vi "F_BSTv2.vi"() -> ()   [LabVIEW 2023]
uses:
  <vilib>/userDefined/High Color/IMAQdx.ctl
  <vilib>/MakerHub/LINX/Public/Peripherals/Digital/Digital Write 1 Chan.vi
  <vilib>/MakerHub/LINX/Public/Peripherals/PWM/PWM Set Duty Cycle 1 Chan.vi
  <vilib>/MakerHub/LINX/Public/Peripherals/Digital/Digital Write N Chans.vi
  <vilib>/MakerHub/LINX/Private/Local IO/LinxDigitalWrite.vi
  <vilib>/MakerHub/LINX/Public/Utilities/Check Channel.vi
  <vilib>/MakerHub/LINX/Public/Utilities/Open Serial.vi
  <vilib>/MakerHub/LINX/Private/Utilties/Generate Error.vi
  <vilib>/MakerHub/LINX/Public/Peripherals/PWM/PWM Set Duty Cycle N Chans.vi
  <vilib>/MakerHub/LINX/LMH-LINX.lvlib
  <vilib>/vision/driver/NI_Vision_Acquisition_Software.lvlib
  <instrlib>/MEDAQLib/MEDAQLib.lvlib
panel:
  in  "Use this stop button to end the test":bool
  in  "?":enum32{"Test Configuration", "Graph"}(tab)
  in  "Click photos in the interval of below cycles":dbl
  in  "Frequency of impact":dbl(knob) step=0.01 scale=0.0..1.0
  in  "No of Cycles":dbl
  in  "Upper limit of duty cycle (%)":dbl(slide) step=0.05 scale=0.0..100.0
  out "Device Name":string
  in  "Serial Port":refnum<visa-resource-name>="N/A"
  in  "Session In":T1
  in  "Images File Path":path
  out "IFM Error Out":string
  in  "Dutycycle File Path":path
  in  "Displacement File Path":path
  out "Image Acquisition Error Out":errorcluster
  out "Serial Communication Error Out":errorcluster
  in  "Force File Path":path
  out "No. of test cycles of dutycycle data saved":dbl
  out "No. of test cycles completed":dbl
  out "Savinng Data":u8(slide) scale=0.0..100.0
  in  "?":bool
  out "?":dbl[](graph)
  out "Right Magnet":dbl
  out "?":waveform(dbl)[](graph)
  out "Left Magnet":dbl
  out "Left Magnet 2":dbl
  out "Right Magnet 2":dbl
  out "?":waveform(dbl)[](graph)
  out "Photo clicked":bool
  out "?":T2(plugin-control)
  out "Test Progress":u8(slide) scale=0.0..100.0
  out "Left magnet max force":dbl
  out "Right magnet max force":dbl
  out "No. of test cycles of displacement data saved":dbl
  out "Savinng Data":u8(slide) scale=0.0..100.0
  in  "?":bool
  # "FBST"
  # "1 - COM PORT OF THE CONTROLLER"
  # "2 - FREQUENCY OF THE SHEAR STRESS"
  # "3 - AMPLITUDE OF THE STRESS"
  # "4 - CYCLES OF THE TEST RUN"
  # "5 - PICTURE DATA SETTINGS"
  # "DUTYCYCLE"
  # "FORCE"
  # "DISPLACEMENT"
  # "VIDEO STREAM"
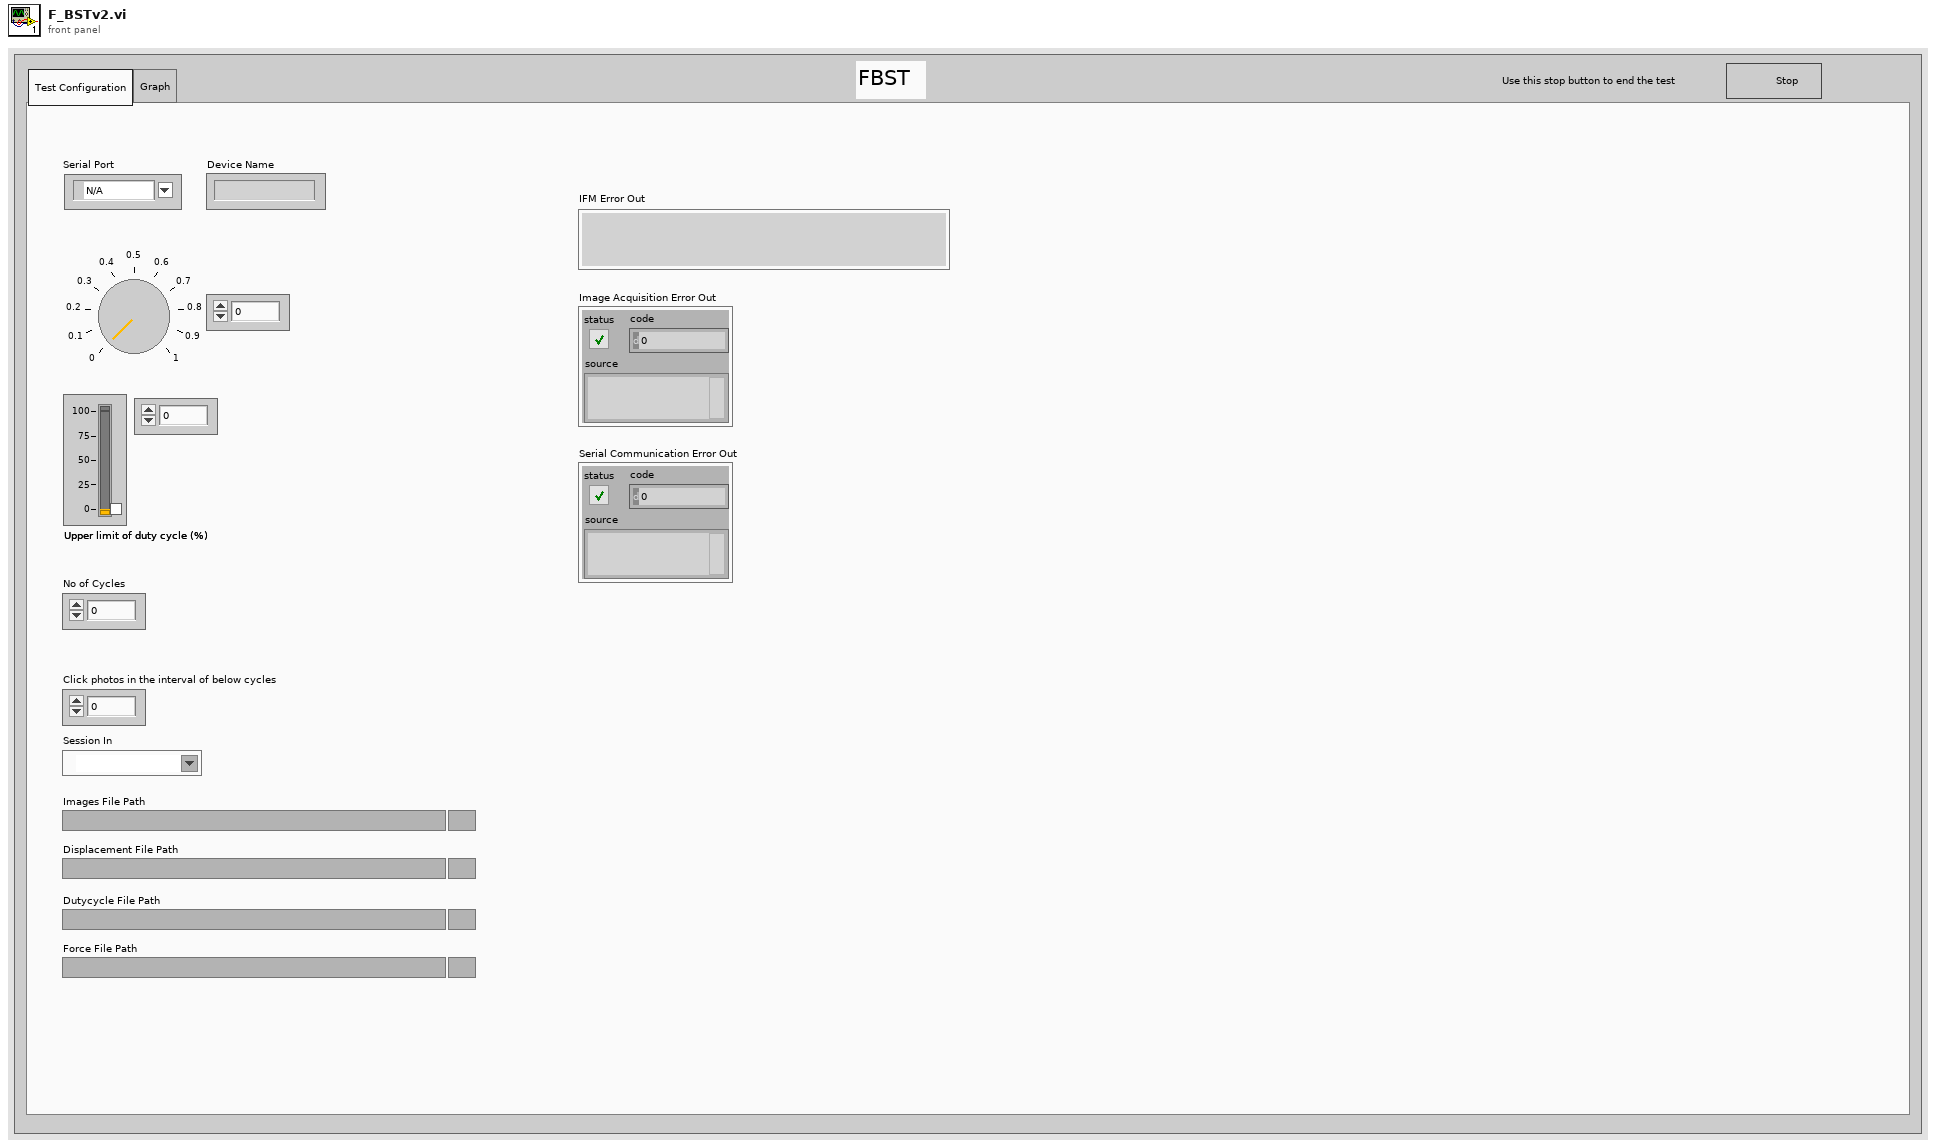
[diagram p1: front panel]
types:
  T1 = typedef "IMAQdx.ctl" = refnum<k21>
  T2 = typedef "IMAQ Image.ctl" = refnum<image>
  T3 = typedef "LMH-LINX.lvlib/LINX Ref.ctl" = cluster{"IO":T4, "Interface":T5, "LINX Device Config":T6}
  T4 = typedef "LMH-LINX.lvlib/Platform.ctl" = enum16{"Remote", "Local"}
  T5 = typedef "LMH-LINX.lvlib/Interface.ctl" = enum16{"Serial", "TCP"}
  T6 = typedef "LMH-LINX.lvlib/Device.lvlib/LINX Device Config.ctl" = cluster{"Interface":T5, "COM Port":refnum<visa-resource-name>, "TCP Configuration":T7, "Device Family":u8, "Device ID":u8, "Device Name":string, "TCP Ref":refnum<k5>, "Channels":T8}
  T7 = typedef "LMH-LINX.lvlib/Device.lvlib/TCP Config.ctl" = cluster{"IP Address":string, "Port":u16}
  T8 = typedef "LMH-LINX.lvlib/Channels.ctl" = cluster{"DI":u8[], "DO":u8[], "AI":u8[], "AO":u8[], "PWM":u8[], "QE":u8[], "UART":u8[], "I2C 2":u8[], "SPI":u8[], "CAN":u8[], "Servo":u8[], "AI Ref (V)":dbl, "AI Resolution (Bits)":u8, "AO Ref (V)":dbl, "AO Resolution (Bits)":u8}
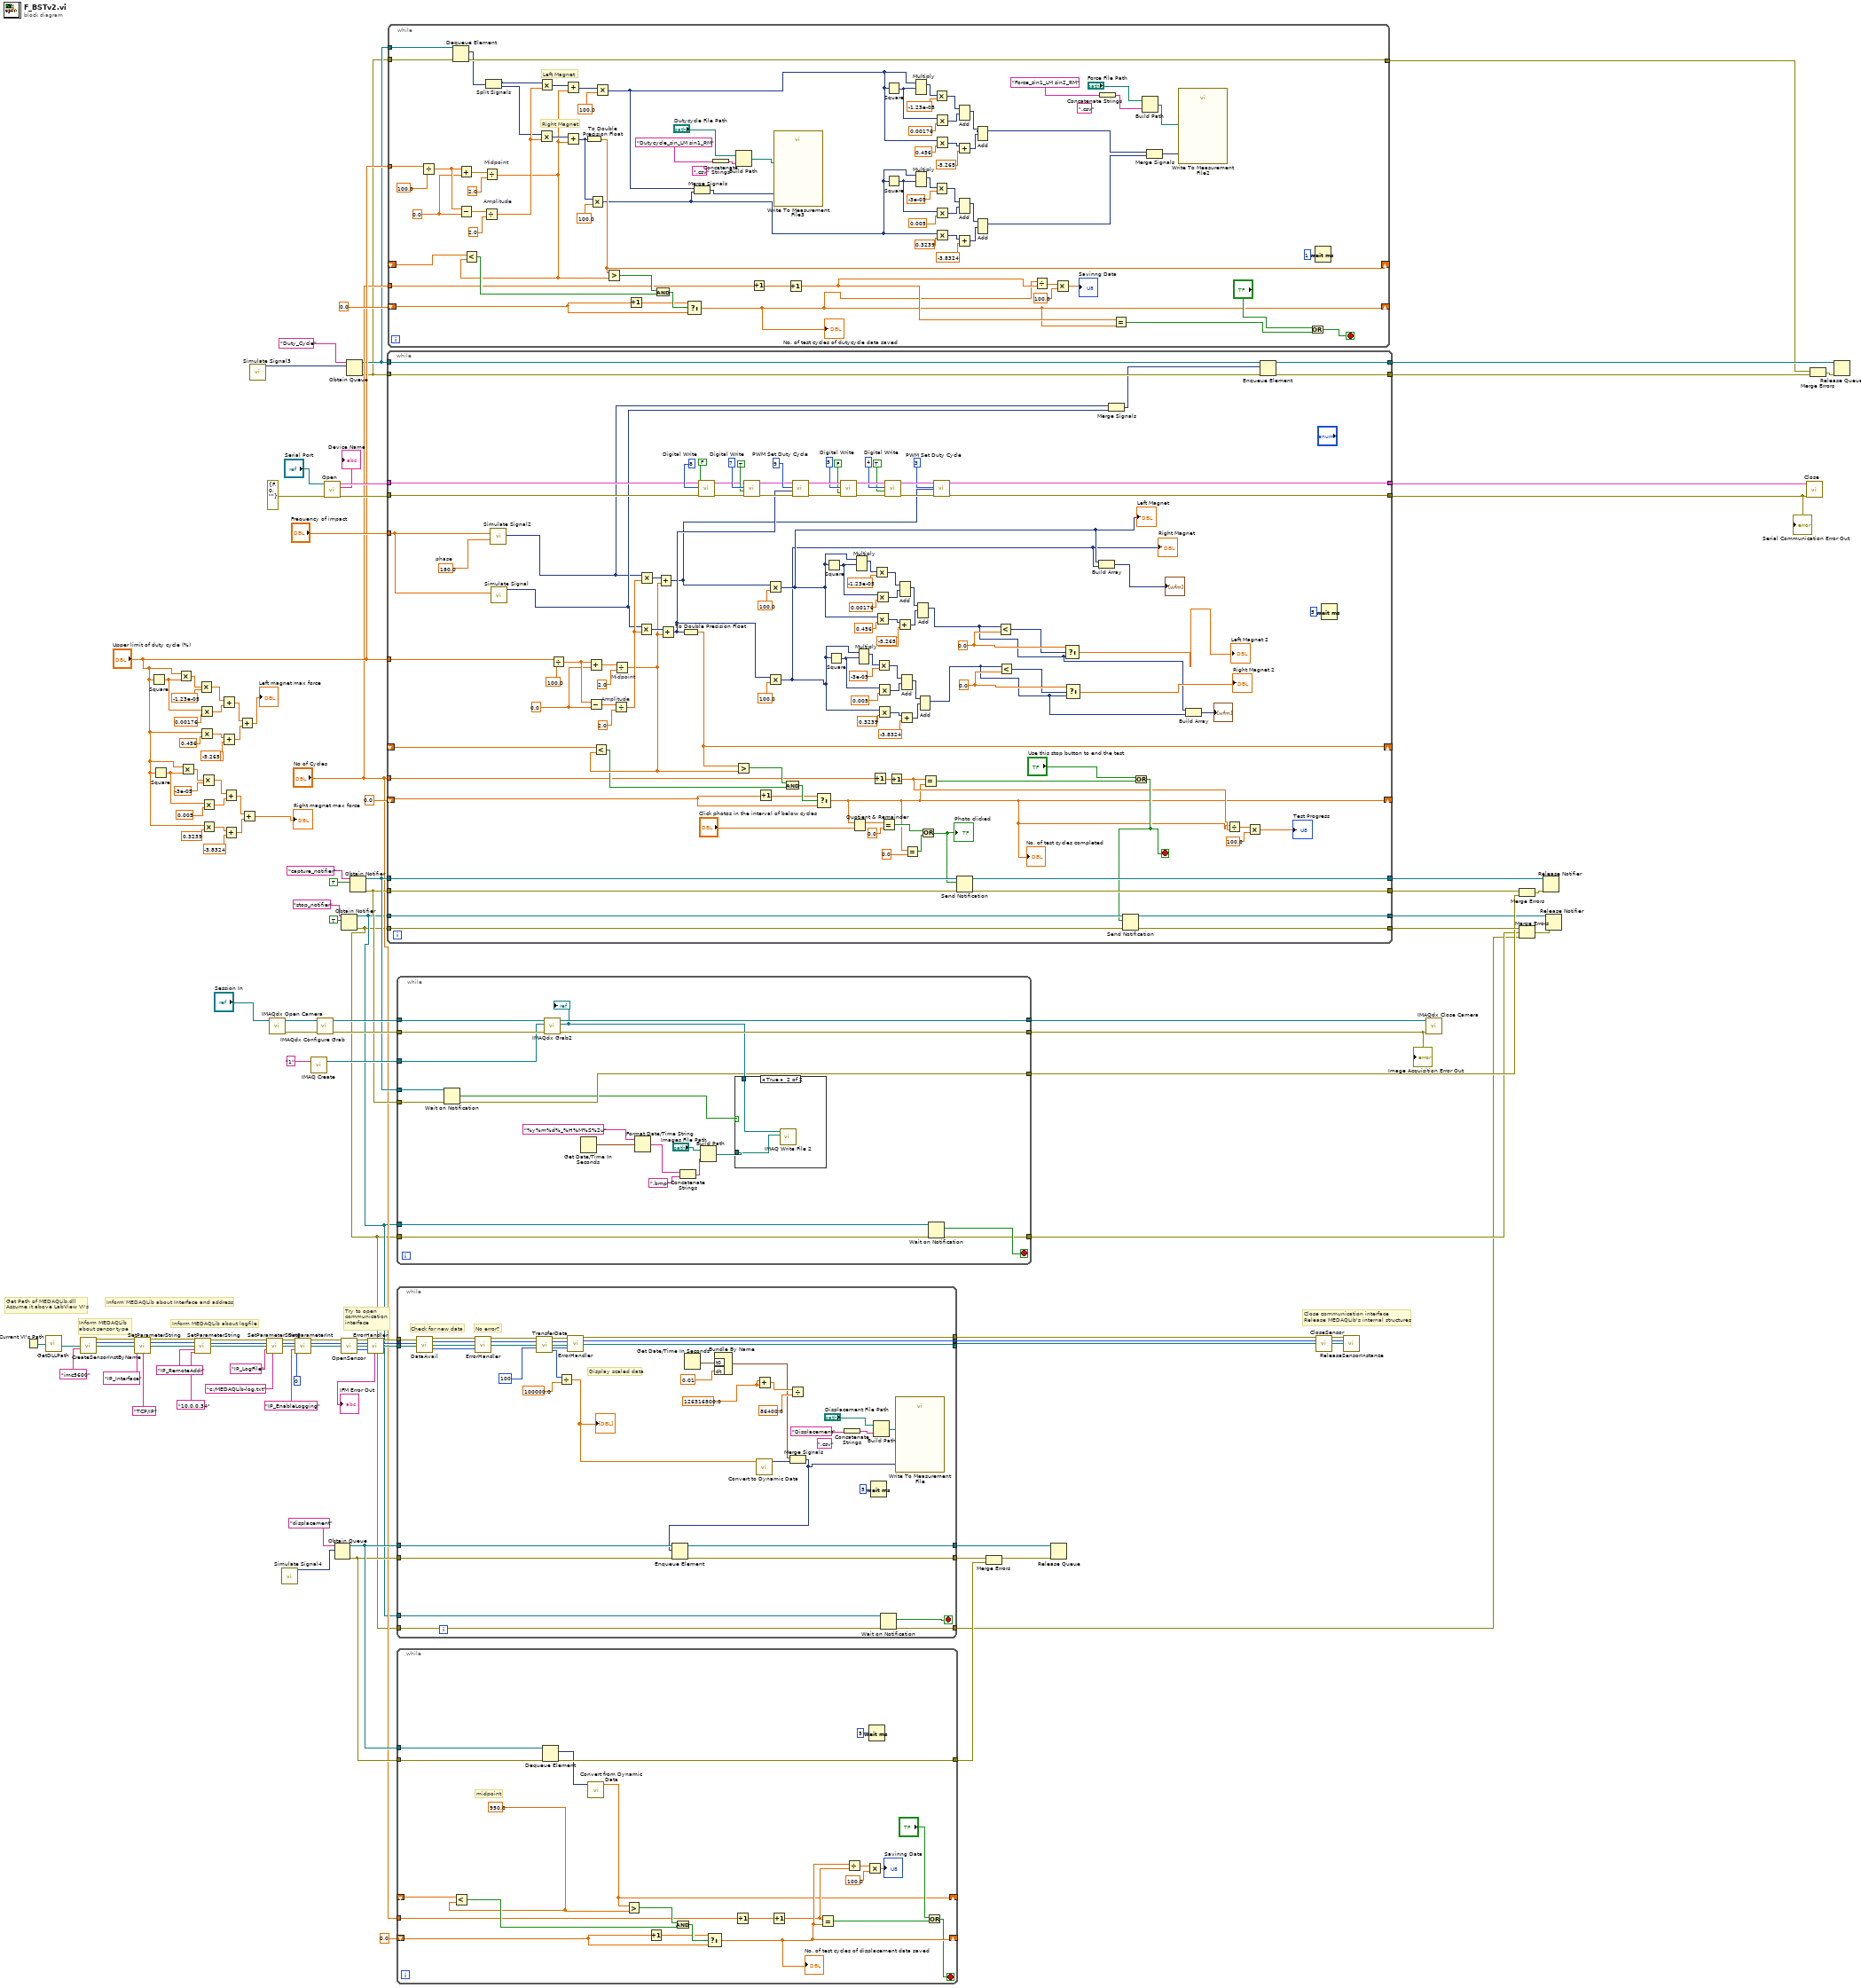
[diagram p0: block diagram]
diagram:
  (unwired) -5.265
  # "Inform MEDAQLib\nabout sensor type"
  # "Get Path of MEDAQLib.dll\nAssume it above LabView VI's"
  # "Try to open\ncommunication\ninterface"
  # "Inform MEDAQLib about logfile"
  # "Inform MEDAQLib about Interface and address"
  # "Close communication interface\nRelease MEDAQLib's internal structures"
  n1 = Current VI's Path() -> (path=w51:path)
  n2 = call <instrlib>:"GetDLLPath.vi"("VI-Path"=w51) -> ("DLL-Path"=w50:path)  [unwired: 10 out]
  n3 = call <instrlib>:"CreateSensorInstByName.vi"("DLL-Path"=w50, "sensor"="imc5600") -> ("Fehler (Ausgang)"=w47:errorcluster, "instanceHandle"=w48:u32, "DLL-Path"=w49:path)  [unwired: 1 in, 10 out]
  n4 = call <instrlib>:"SetParameterString.vi"("Fehler (Eingang, kein Fehler)"=w47, "instanceHandle"=w48, "DLL-Path"=w49, "paramName"="IP_Interface", "paramValue"="TCP/IP") -> ("Fehler (Ausgang)"=w43:errorcluster, "instanceHandle"=w42:u32, "DLL-Path"=w41:path)  [unwired: 8 out]
  n5 = Square(x="Upper limit of duty cycle (%)") -> (x^2=w33:dbl)
  n6 = Square(x="Upper limit of duty cycle (%)") -> (x^2=w22:dbl)
  n7 = Multiply(x="Upper limit of duty cycle (%)", y=w33) -> (x*y=w36:dbl)
  n8 = Multiply(x="Upper limit of duty cycle (%)", y=w22) -> (x*y=w25:dbl)
  n9 = call <instrlib>:"SetParameterString.vi"("Fehler (Eingang, kein Fehler)"=w43, "instanceHandle"=w42, "DLL-Path"=w41, "paramName"="IP_RemoteAddr", "paramValue"="10.0.0.34") -> ("Fehler (Ausgang)"=w85:errorcluster, "instanceHandle"=w84:u32, "DLL-Path"=w83:path)  [unwired: 8 out]
  n10 = Multiply(x=w36, y=-1.23e-05) -> (x*y=w31:dbl)
  n11 = Multiply(x=w33, y=0.00176) -> (x*y=w30:dbl)
  n12 = Multiply(x="Upper limit of duty cycle (%)", y=0.456) -> (x*y=w29:dbl)
  n13 = Multiply(x=w25, y=-3e-05) -> (x*y=w20:dbl)
  n14 = Multiply(x=w22, y=0.005) -> (x*y=w19:dbl)
  n15 = Multiply(x="Upper limit of duty cycle (%)", y=0.3239) -> (x*y=w18:dbl)
  n16 = Add(x=w31, y=w30) -> (x+y=w27:dbl)
  n17 = Add(x=w29, y=-5.265) -> (x+y=w26:dbl)
  n18 = Add(x=w20, y=w19) -> (x+y=w16:dbl)
  n19 = Add(x=w18, y=-3.8324) -> (x+y=w15:dbl)
  n20 = Add(x=w27, y=w26) -> (x+y=→"Left magnet max force":dbl)
  n21 = Add(x=w16, y=w15) -> (x+y=→"Right magnet max force":dbl)
  n22 = call "Simulate Signal3"() -> ("Sine"=w53:dynamicdata)  [unwired: 14 in, 1 out]
  n23 = call <instrlib>:"SetParameterString.vi"("Fehler (Eingang, kein Fehler)"=w85, "instanceHandle"=w84, "DLL-Path"=w83, "paramName"="IP_LogFile", "paramValue"="c:/MEDAQLib-log.txt") -> ("Fehler (Ausgang)"=w80:errorcluster, "instanceHandle"=w79:u32, "DLL-Path"=w78:path)  [unwired: 8 out]
  n24 = call <vilib>:"IMAQdx Open Camera.vi"("Session In"="Session In") -> ("error out"=w100:errorcluster, "Session Out"=w101:T1)  [unwired: 9 in]
  n25 = call "Simulate Signal4"() -> ("Sine"=w1:dynamicdata)  [unwired: 14 in, 1 out]
  n26 = call <instrlib>:"SetParameterInt.vi"("Fehler (Eingang, kein Fehler)"=w80, "instanceHandle"=w79, "DLL-Path"=w78, "paramName"="IP_EnableLogging", "paramValue"=0) -> ("Fehler (Ausgang)"=w75:errorcluster, "instanceHandle"=w74:u32, "DLL-Path"=w73:path)  [unwired: 8 out]
  n27 = call "IMAQ Create"("Image Name"="1") -> ("New Image"=w96:T2)  [unwired: 4 in, 1 out]
  n28 = call <vilib>:"IMAQdx Configure Grab.vi"("error in"=w100, "Session In"=w101) -> ("error out"=w97:errorcluster, "Session Out"=w98:T1)  [unwired: 8 in]
  n29 = call-poly <vilib>:"Open.vi"("Error In"=errorcluster {"status"=FALSE, "code"=0, "source"=""}, "Serial Port"="Serial Port") -> ("Error Out"=w116:errorcluster, "Device Name"=→"Device Name":string, "LINX Resource"=w117:T3)  [unwired: 7 in]
  n30 = Obtain Queue(name (unnamed)="displacement", element data type=w1) -> (queue out=w12:refnum<queue>, error out=w11:errorcluster)  [unwired: 3 in, 1 out]
  n31 = Obtain Notifier(name (unnamed)="stop_notifier", notification data type=TRUE) -> (notifier out=w4:refnum<notifier>, error out=w3:errorcluster)  [unwired: 2 in, 1 out]
  n32 = call <instrlib>:"OpenSensor.vi"("Fehler (Eingang, kein Fehler)"=w75, "instanceHandle"=w74, "DLL-Path"=w73) -> ("Fehler (Ausgang)"=w71:errorcluster, "instanceHandle"=w70:u32, "DLL-Path"=w69:path, "ERR_CODE"=w72:i32)  [unwired: 9 out]
  n33 = Obtain Queue(name (unnamed)="Duty_Cycle", element data type=w53) -> (queue out=w6:refnum<queue>, error out=w5:errorcluster)  [unwired: 3 in, 1 out]
  n34 = Obtain Notifier(name (unnamed)="capture_notifier", notification data type=TRUE) -> (notifier out=w91:refnum<notifier>, error out=w90:errorcluster)  [unwired: 2 in, 1 out]
  n35 = call <instrlib>:"ErrorHandler.vi"("Fehler (Eingang, kein Fehler)"=w71, "instanceHandle"=w70, "DLL-Path"=w69, "ERR_CODE"=w72) -> ("Fehler (Ausgang)"=w67:errorcluster, "instanceHandle"=w66:u32, "DLL-Path"=w65:path, "errText"=→"IFM Error Out":string)  [unwired: 8 out]
  n36 = while {
    tunnel: w117 -> [w205]
    tunnel: w116 -> [w235]
    tunnel: [w199] -> w115
    tunnel: [w198] -> w114
    shift-right: [w160] -> _
    shift-left: 0.0 -> [w182]
    shift-right: [w178] -> _
    shift-left: _ -> [w204]
    tunnel: w91 -> [w196]
    tunnel: [w195] -> w111
    tunnel: w90 -> [w194]
    tunnel: [w193] -> w105
    tunnel: w4 -> [w186]
    tunnel: [w185] -> w61
    tunnel: w3 -> [w174]
    tunnel: [w184] -> w104
    tunnel: w6 -> [w172]
    tunnel: w5 -> [w171]
    tunnel: [w175] -> w58
    tunnel: [w170] -> w60
    tunnel: "No of Cycles" -> [w168]
    tunnel: "Upper limit of duty cycle (%)" -> [w167]
    tunnel: "Frequency of impact" -> [w166]
    stop <- w180 stop-if-true
    w127 = 0.0 ("y")
    w130 = 0.0 ("y")
    (unwired) -5.265
    w176 = 0.0 ("y")
    w181 = 180.0  # phase
    n37 = call "Simulate Signal2"("Frequency"=w166, "Phase"=w181) -> ("Sine"=w120:dynamicdata)  [unwired: 12 in, 1 out]
    n38 = call "Simulate Signal"("Frequency"=w166) -> ("Sine"=w161:dynamicdata)  [unwired: 13 in, 1 out]
    n39 = Divide(x=w167, y=100.0) -> (x/y=w208:dbl)
    n40 = Add(x=w208, y=w176) -> (x+y=w214:dbl)
    n41 = Subtract(x=w208, y=w176) -> (x-y=w212:dbl)
    n42 = Divide "Amplitude"(x=w212, y=2.0) -> (x/y=w206:dbl)
    n43 = Divide "Midpoint"(x=w214, y=2.0) -> (x/y=w203:dbl)
    n44 = Less?(x=w204, y=w203) -> (x < y?=w201:bool)
    n45 = Multiply(x=w161, y=w206) -> (x*y=w210:dynamicdata)
    n46 = Multiply(x=w120, y=w206) -> (x*y=w207:dynamicdata)
    n47 = Add(x=w207, y=w203) -> (x+y=w144:dynamicdata)
    n48 = Add(x=w210, y=w203) -> (x+y=w145:dynamicdata)
    n49 = To Double Precision Float(number=w145) -> (double precision float=w178:dbl)
    n50 = call-poly <vilib>:"Digital Write.vi"("Error In"=w235, "Output Value"=FALSE, "DO Channel"=u8 8, "LINX Resource"=w205) -> ("Error Out"=w230:errorcluster, "LINX Resource"=w231:T3)  [unwired: 6 in]
    n51 = Greater?(x=w178, y=w203) -> (0:w202:bool)
    n52 = call-poly <vilib>:"Digital Write.vi"("Error In"=w230, "Output Value"=TRUE, "DO Channel"=u8 7, "LINX Resource"=w231) -> ("Error Out"=w226:errorcluster, "LINX Resource"=w227:T3)  [unwired: 6 in]
    n53 = Increment(x=w182) -> (x+1=w197:dbl)
    n54 = Multiply(x=w144, y=100.0) -> (x*y=w143:dynamicdata)
    "Left Magnet" <- w143
    n55 = Multiply(x=w145, y=100.0) -> (x*y=w131:dynamicdata)
    "Right Magnet" <- w131
    n56 = And(x=w202, y=w201) -> (x .and. y?=w200:bool)
    n57 = call-poly <vilib>:"PWM Set Duty Cycle.vi"("Error In"=w226, "Duty Cycle (0-1)"=w145, "PWM Channel"=u8 9, "LINX Resource"=w227) -> ("Error Out"=w220:errorcluster, "LINX Resource"=w221:T3)  [unwired: 6 in]
    n58 = Select(t=w197, s=w200, f=w182) -> (s? t:f=w160:dbl)
    "No. of test cycles completed" <- w160
    n59 = Square(x=w143) -> (x^2=w154:dynamicdata)
    n60 = Square(x=w131) -> (x^2=w139:dynamicdata)
    n61 = call-poly <vilib>:"Digital Write.vi"("Error In"=w220, "Output Value"=FALSE, "DO Channel"=u8 5, "LINX Resource"=w221) -> ("Error Out"=w223:errorcluster, "LINX Resource"=w222:T3)  [unwired: 6 in]
    n62 = Quotient & Remainder(x=w160, y="Click photos in the interval of below cycles") -> (x-y*floor(x/y)=w192:dbl)  [unwired: 1 out]
    n63 = Multiply(1:w154, 2:w143) -> (0:w157:dynamicdata)  [unwired: 1 in, 1 out]
    n64 = Multiply(1:w139, 2:w131) -> (0:w142:dynamicdata)  [unwired: 1 in, 1 out]
    n65 = Increment(x=w168) -> (x+1=w173:dbl)
    n66 = Multiply(x=w157, y=-1.23e-05) -> (x*y=w151:dynamicdata)
    n67 = Multiply(x=w154, y=0.00176) -> (x*y=w150:dynamicdata)
    n68 = Multiply(x=w143, y=0.456) -> (x*y=w149:dynamicdata)
    n69 = Multiply(x=w142, y=-3e-05) -> (x*y=w137:dynamicdata)
    n70 = Multiply(x=w139, y=0.005) -> (x*y=w136:dynamicdata)
    n71 = Multiply(x=w131, y=0.3239) -> (x*y=w135:dynamicdata)
    n72 = Equal?(x=w192, y=0.0) -> (x = y?=w188:bool)
    n73 = call-poly <vilib>:"Digital Write.vi"("Error In"=w223, "Output Value"=TRUE, "DO Channel"=u8 4, "LINX Resource"=w222) -> ("Error Out"=w225:errorcluster, "LINX Resource"=w224:T3)  [unwired: 6 in]
    n74 = Increment(x=w173) -> (x+1=w162:dbl)
    n75 = Add(1:w150, 2:w151) -> (0:w147:dynamicdata)  [unwired: 1 in, 1 out]
    n76 = Add(x=w149, y=-5.265) -> (x+y=w146:dynamicdata)
    n77 = Add(1:w136, 2:w137) -> (0:w133:dynamicdata)  [unwired: 1 in, 1 out]
    n78 = Add(x=w135, y=-3.8324) -> (x+y=w132:dynamicdata)
    n79 = Equal?(x=w160, y=0.0) -> (x = y?=w189:bool)
    n80 = Add(1:w146, 2:w147) -> (0:w124:dynamicdata)  [unwired: 1 in, 1 out]
    n81 = Add(1:w132, 2:w133) -> (0:w123:dynamicdata)  [unwired: 1 in, 1 out]
    n82 = Or(x=w188, y=w189) -> (x .or. y?=w187:bool)
    "Photo clicked" <- w187
    n83 = Equal?(x=w162, y=w160) -> (x = y?=w179:bool)
    n84 = call-poly <vilib>:"PWM Set Duty Cycle.vi"("Error In"=w225, "Duty Cycle (0-1)"=w144, "PWM Channel"=u8 3, "LINX Resource"=w224) -> ("Error Out"=w198:errorcluster, "LINX Resource"=w199:T3)  [unwired: 6 in]
    n85 = Send Notification(notification=w187, notifier=w196, error in (no error)=w194) -> (notifier out=w195:refnum<notifier>, error out=w193:errorcluster)
    n86 = Less?(x=w124, y=w130) -> (x < y?=w129:dynamicdata)
    n87 = Less?(x=w123, y=w127) -> (x < y?=w126:dynamicdata)
    n88 = Select(t=w130, s=w129, f=w124) -> (s? t:f=→"Left Magnet 2":dbl)
    n89 = Select(t=w127, s=w126, f=w123) -> (s? t:f=→"Right Magnet 2":dbl)
    n90 = Build Array(w143, w131) -> (→"?":dynamicdata[])
    n91 = Merge Signals(w120, w161) -> (w159:dynamicdata)
    n92 = Or(x="Use this stop button to end the test", y=w179) -> (x .or. y?=w180:bool)
    n93 = Send Notification(notification=w180, notifier=w186, error in (no error)=w174) -> (notifier out=w185:refnum<notifier>, error out=w184:errorcluster)
    n94 = Build Array(w124, w123) -> (→"?":dynamicdata[])
    n95 = Divide(x=w160, y=w162) -> (x/y=w165:dbl)
    n96 = Multiply(x=w165, y=100.0) -> (x*y=→"Test Progress":dbl)
    n97 = Enqueue Element(queue=w172, element=w159, error in (no error)=w171) -> (queue out=w170:refnum<queue>, error out=w175:errorcluster)  [unwired: 1 in, 1 out]
    n98 = Wait (ms)(milliseconds to wait=u32 5) -> ()  [unwired: 1 out]
  }
  "Serial Communication Error Out" <- w114
  n99 = while {
    tunnel: "No of Cycles" -> [w297]
    tunnel: "Upper limit of duty cycle (%)" -> [w295]
    tunnel: w6 -> [w294]
    tunnel: w5 -> [w293]
    tunnel: [w292] -> w56
    shift-right: [w237] -> _
    shift-left: 0.0 -> [w291]
    shift-right: [w283] -> _
    shift-left: _ -> [w290]
    stop <- w281 stop-if-true
    (unwired) ".csv"
    (unwired) ".csv"
    w296 = 0.0 ("y")
    # "Right Magnet"
    # "Left Magnet"
    n100 = Divide(x=w295, y=100.0) -> (x/y=w305:dbl)
    n101 = Dequeue Element(queue=w294, error in (no error)=w293) -> (element=w278:dynamicdata, error out=w292:errorcluster)  [unwired: 1 in, 2 out]
    n102 = Add(x=w305, y=w296) -> (x+y=w311:dbl)
    n103 = Subtract(x=w305, y=w296) -> (x-y=w309:dbl)
    n104 = Divide "Amplitude"(x=w309, y=2.0) -> (x/y=w303:dbl)
    n105 = Divide "Midpoint"(x=w311, y=2.0) -> (x/y=w282:dbl)
    n106 = Less?(x=w290, y=w282) -> (x < y?=w301:bool)
    n107 = Split Signals(w278) -> (w277:dynamicdata, w272:dynamicdata)  [unwired: 2 in]
    n108 = Multiply(x=w272, y=w303) -> (x*y=w307:dynamicdata)
    n109 = Multiply(x=w277, y=w303) -> (x*y=w304:dynamicdata)
    n110 = Add(x=w304, y=w282) -> (x+y=w274:dynamicdata)
    n111 = Add(x=w307, y=w282) -> (x+y=w273:dynamicdata)
    n112 = To Double Precision Float(number=w273) -> (double precision float=w283:dbl)
    n113 = Multiply(x=w273, y=100.0) -> (x*y=w240:dynamicdata)
    n114 = Multiply(x=w274, y=100.0) -> (x*y=w239:dynamicdata)
    n115 = Greater?(x=w283, y=w282) -> (0:w302:bool)
    n116 = Increment(x=w291) -> (x+1=w299:dbl)
    n117 = And(x=w302, y=w301) -> (x .and. y?=w300:bool)
    n118 = Select(t=w299, s=w300, f=w291) -> (s? t:f=w237:dbl)
    "No. of test cycles of dutycycle data saved" <- w237
    n119 = Merge Signals(w239, w240) -> (w270:dynamicdata)
    n120 = Concatenate Strings("Dutycycle_sin_LM sin1_RM" ("time format string (%c)")) -> (w285:string)
    n121 = Build Path(base path="Dutycycle File Path", name or relative path=w285) -> (appended path=w271:path)
    n122 = Increment(x=w297) -> (x+1=w298:dbl)
    n123 = call "Write To Measurement File3"("Signals"=w270, "Filename"=w271) -> ()  [unwired: 15 in, 3 out]
    n124 = Increment(x=w298) -> (x+1=w238:dbl)
    n125 = Square(x=w239) -> (x^2=w251:dynamicdata)
    n126 = Square(x=w240) -> (x^2=w262:dynamicdata)
    n127 = Multiply(1:w251, 2:w239) -> (0:w254:dynamicdata)  [unwired: 1 in, 1 out]
    n128 = Multiply(1:w262, 2:w240) -> (0:w265:dynamicdata)  [unwired: 1 in, 1 out]
    n129 = Multiply(x=w254, y=-1.23e-05) -> (x*y=w249:dynamicdata)
    n130 = Multiply(x=w265, y=-3e-05) -> (x*y=w260:dynamicdata)
    n131 = Multiply(x=w251, y=0.00176) -> (x*y=w248:dynamicdata)
    n132 = Multiply(x=w239, y=0.456) -> (x*y=w247:dynamicdata)
    n133 = Multiply(x=w262, y=0.005) -> (x*y=w259:dynamicdata)
    n134 = Multiply(x=w240, y=0.3239) -> (x*y=w258:dynamicdata)
    n135 = Add(1:w248, 2:w249) -> (0:w245:dynamicdata)  [unwired: 1 in, 1 out]
    n136 = Add(x=w247, y=-5.265) -> (x+y=w244:dynamicdata)
    n137 = Add(1:w259, 2:w260) -> (0:w256:dynamicdata)  [unwired: 1 in, 1 out]
    n138 = Add(x=w258, y=-3.8324) -> (x+y=w255:dynamicdata)
    n139 = Add(1:w244, 2:w245) -> (0:w243:dynamicdata)  [unwired: 1 in, 1 out]
    n140 = Add(1:w255, 2:w256) -> (0:w242:dynamicdata)  [unwired: 1 in, 1 out]
    n141 = Divide(x=w237, y=w238) -> (x/y=w288:dbl)
    n142 = Multiply(x=w288, y=100.0) -> (x*y=→"Savinng Data":dbl)
    n143 = Concatenate Strings("Force_sin1_LM sin2_RM" ("time format string (%c)")) -> (w268:string)
    n144 = Equal?(x=w238, y=w237) -> (x = y?=w236:bool)
    n145 = Build Path(base path="Force File Path", name or relative path=w268) -> (appended path=w266:path)
    n146 = Merge Signals(w243, w242) -> (w241:dynamicdata)
    n147 = call "Write To Measurement File2"("Signals"=w241, "Filename"=w266) -> ()  [unwired: 15 in, 3 out]
    n148 = Or(x="?", y=w236) -> (x .or. y?=w281:bool)
    n149 = Wait (ms)(milliseconds to wait=u32 1) -> ()  [unwired: 1 out]
  }
  n150 = while {
    tunnel: w67 -> [w342]
    tunnel: w66 -> [w341]
    tunnel: w65 -> [w340]
    tunnel: [w339] -> w64
    tunnel: [w338] -> w63
    tunnel: [w337] -> w62
    tunnel: [w335] -> w2
    tunnel: w12 -> [w331]
    tunnel: w11 -> [w334]
    tunnel: [w333] -> w40
    tunnel: [w332] -> w37
    tunnel: w4 -> [w327]
    tunnel: w3 -> [w326]
    stop <- w336 stop-if-true
    (unwired) ".csv"
    w317 = 126316800.0 ("y")
    # "Display scaled data"
    # "No error?"
    # "Check for new data"
    n151 = call <instrlib>:"DataAvail.vi"("Fehler (Eingang, kein Fehler)"=w342, "instanceHandle"=w341, "DLL-Path"=w340) -> ("Fehler (Ausgang)"=w353:errorcluster, "instanceHandle"=w351:u32, "DLL-Path"=w349:path, "ERR_CODE"=w347:i32)  [unwired: 9 out]
    n152 = call <instrlib>:"ErrorHandler.vi"("Fehler (Eingang, kein Fehler)"=w353, "instanceHandle"=w351, "DLL-Path"=w349, "ERR_CODE"=w347) -> ("Fehler (Ausgang)"=w352:errorcluster, "instanceHandle"=w350:u32, "DLL-Path"=w348:path)  [unwired: 9 out]
    n153 = call <instrlib>:"TransferData.vi"("Fehler (Eingang, kein Fehler)"=w352, "instanceHandle"=w350, "DLL-Path"=w348, "maxValues"=100) -> ("Fehler (Ausgang)"=w346:errorcluster, "instanceHandle"=w345:u32, "DLL-Path"=w344:path, "ERR_CODE"=w343:i32, "rawData"=w329:i32[])  [unwired: 7 out]
    n154 = Divide(x=w329, y=100000.0) -> (x/y=w323:dbl[])
    "?" <- w323
    n155 = call <instrlib>:"ErrorHandler.vi"("Fehler (Eingang, kein Fehler)"=w346, "instanceHandle"=w345, "DLL-Path"=w344, "ERR_CODE"=w343) -> ("Fehler (Ausgang)"=w339:errorcluster, "instanceHandle"=w338:u32, "DLL-Path"=w337:path)  [unwired: 9 out]
    n156 = Get Date/Time In Seconds() -> (seconds since 1Jan1904=w315:timestamp)
    n157 = Bundle By Name("t0"=w315, "dt"=0.01) -> (w313:waveform(dbl))  [unwired: 1 in]
    n158 = call "Convert to Dynamic Data"("Array"=w323) -> ("Dynamic Data Type"=w322:dynamicdata)  [unwired: 3 in]
    n159 = Add(x=w317, y=w317) -> (x+y=w324:dbl)
    n160 = Divide(x=w324, y=86400.0) -> ()  [unwired: 1 out]
    n161 = Merge Signals(w313, w322) -> (w312:dynamicdata)
    n162 = Enqueue Element(queue=w331, element=w312, error in (no error)=w334) -> (queue out=w333:refnum<queue>, error out=w332:errorcluster)  [unwired: 1 in, 1 out]
    n163 = Concatenate Strings("Displacement" ("time format string (%c)")) -> (w319:string)
    n164 = Wait (ms)(milliseconds to wait=u32 5) -> ()  [unwired: 1 out]
    n165 = Build Path(base path="Displacement File Path", name or relative path=w319) -> (appended path=w321:path)
    n166 = Wait on Notification(notifier=w327, error in (no error)=w326) -> (notification=w336:bool, error out=w335:errorcluster)  [unwired: 2 in, 2 out]
    n167 = call "Write To Measurement File"("Signals"=w312, "Filename"=w321) -> ()  [unwired: 15 in, 3 out]
  }
  n168 = while {
    tunnel: w12 -> [w376]
    tunnel: w11 -> [w375]
    tunnel: [w374] -> w10
    shift-right: [w358] -> _
    shift-left: _ -> [w362]
    shift-right: [w366] -> _
    shift-left: 0.0 ("y") -> [w369]
    tunnel: "No of Cycles" -> [w357]
    stop <- w360 stop-if-true
    w361 = 950.0 ("y")
    # "midpoint"
    n169 = Less?(x=w362, y=w361) -> (x < y?=w372:bool)
    n170 = Dequeue Element(queue=w376, error in (no error)=w375) -> (element=w354:dynamicdata, error out=w374:errorcluster)  [unwired: 1 in, 2 out]
    n171 = call "Convert from Dynamic Data"("Dynamic Data Type"=w354) -> ("Scalar"=w358:dbl)  [unwired: 3 in]
    n172 = Greater?(x=w358, y=w361) -> (0:w373:bool)
    n173 = Increment(x=w369) -> (x+1=w370:dbl)
    n174 = And(x=w373, y=w372) -> (x .and. y?=w371:bool)
    n175 = Select(t=w370, s=w371, f=w369) -> (s? t:f=w366:dbl)
    "No. of test cycles of displacement data saved" <- w366
    n176 = Increment(x=w357) -> (x+1=w356:dbl)
    n177 = Increment(x=w356) -> (x+1=w359:dbl)
    n178 = Equal?(x=w359, y=w366) -> (x = y?=w364:bool)
    n179 = Divide(x=w366, y=w359) -> (x/y=w367:dbl)
    n180 = Multiply(x=w367, y=100.0) -> (x*y=→"Savinng Data":dbl)
    n181 = Wait (ms)(milliseconds to wait=u32 5) -> ()  [unwired: 1 out]
    n182 = Or(x="?", y=w364) -> (x .or. y?=w360:bool)
  }
  n183 = while {
    tunnel: w91 -> [w397]
    tunnel: w90 -> [w396]
    tunnel: w98 -> [w388]
    tunnel: w97 -> [w387]
    tunnel: w96 -> [w386]
    tunnel: [w385] -> w95
    tunnel: [w384] -> w94
    tunnel: w4 -> [w382]
    tunnel: w3 -> [w381]
    tunnel: [w379] -> w93
    tunnel: [w378] -> w92
    stop <- w380 stop-if-true
    n184 = Wait on Notification(notifier=w397, error in (no error)=w396) -> (notification=w377:bool, error out=w379:errorcluster)  [unwired: 2 in, 2 out]
    n185 = call <vilib>:"IMAQdx Grab2.vi"("error in"=w387, "Image In"=w386, "Session In"=w388) -> ("error out"=w384:errorcluster, "Image Out"=w383:T2, "Session Out"=w385:T1)  [unwired: 5 in, 1 out]
    "?" <- w383
    n186 = Get Date/Time In Seconds() -> (seconds since 1Jan1904=w393:timestamp)
    n187 = Format Date/Time String(time format string (%c)="%y%m%d%_%H%M%S%2u", seconds (now)=w393) -> (date/time string=w392:string)  [unwired: 1 in]
    n188 = Concatenate Strings(w392, ".bmp") -> (w394:string)
    n189 = Build Path(base path="Images File Path", name or relative path=w394) -> (appended path=w389:path)
    n190 = case shown="True" w377 {
      tunnel: w383 -> [_ w399]
      tunnel: w389 -> [_ w398]
      frame False {
      }
      frame True {
        n191 = call-poly "IMAQ Write File 2"("File Path"=w398, "Image"=w399) -> ()  [unwired: 8 in, 2 out]
      }
    }
    n192 = Wait on Notification(notifier=w382, error in (no error)=w381) -> (notification=w380:bool, error out=w378:errorcluster)  [unwired: 2 in, 2 out]
  }
  "Image Acquisition Error Out" <- w94
  n193 = Merge Errors(w37, w10) -> (w38:errorcluster)
  n194 = Release Queue(queue=w40, error in (no error)=w38) -> ()  [unwired: 1 in, 3 out]
  n195 = call <instrlib>:"CloseSensor.vi"("Fehler (Eingang, kein Fehler)"=w64, "instanceHandle"=w63, "DLL-Path"=w62) -> ("Fehler (Ausgang)"=w89:errorcluster, "instanceHandle"=w88:u32, "DLL-Path"=w87:path)  [unwired: 10 out]
  n196 = call <instrlib>:"ReleaseSensorInstance.vi"("Fehler (Eingang, kein Fehler)"=w89, "instanceHandle"=w88, "DLL-Path"=w87) -> ()  [unwired: 13 out]
  n197 = call <vilib>:"IMAQdx Close Camera.vi"("error in"=w94, "Session In"=w95) -> ()  [unwired: 9 in, 1 out]
  n198 = Merge Errors(w105, w93) -> (w106:errorcluster)
  n199 = Merge Errors(w104, w92, w2) -> (w103:errorcluster)
  n200 = Release Notifier(notifier=w111, error in (no error)=w106) -> ()  [unwired: 1 in, 3 out]
  n201 = Release Notifier(notifier=w61, error in (no error)=w103) -> ()  [unwired: 1 in, 3 out]
  n202 = call <vilib>:"Close.vi"("Error In"=w114, "LINX Resource"=w115) -> ()  [unwired: 9 in, 1 out]
  n203 = Merge Errors(w56, w58) -> (w59:errorcluster)
  n204 = Release Queue(queue=w60, error in (no error)=w59) -> ()  [unwired: 1 in, 3 out]
